vi "Test Process No Process Errors Through Basic Lifecycle.vi"(8 "error in (no error)":errorcluster, 11 "Process Test In":refnum<class "Process Dev Test.lvclass">) -> (0 "error out":errorcluster, 3 "Process Test Out":refnum<class "Process Dev Test.lvclass">)   [LabVIEW 2020, in "Process Dev Test.lvclass"]
uses:
  Mock Error Handler/Mock Error Handler.lvclass
  C:/Git/astemes-triarc-framework/source/Framework/Error Handler Interface/Error Handler Interface.lvclass
  Framework/Process/Process.lvclass/Process.ctl
  <vilib>/Astemes/LUnit/Test Case.lvclass/Test Case.ctl
  <vilib>/Astemes/LUnit/LUnit Assertion Result.lvclass/LUnit Assertion Result.ctl
  <vilib>/Astemes/LUnit/LUnit Test Case Result.lvclass/LUnit Test Case Result.ctl
  <vilib>/Astemes/LUnit/LUnit Method Result.lvclass/LUnit Method Result.ctl
  Framework/Process/Protected/Messaging/Enqueue Message.vi
  Framework/Process/Public/Lifecycle/Get Lifecycle State.vi
  Framework/Process/Private/SubVIs/Wait for finish.vi
  Framework/Process/Private/SubVIs/Set Lifecycle State.vi
  <vilib>/Astemes/LUnit/Palette/Pass.vi
  <vilib>/Astemes/LUnit/Palette/Fail.vi
  <vilib>/Astemes/LUnit/Set Assertion Type.vi
  Framework/Process/Private/SubVIs/Handle Debug Data.vi
  <vilib>/Utility/error.llb/Clear Errors.vi
  <vilib>/Astemes/LUnit/Add test result.vi
  <vilib>/Astemes/LUnit/LUnit Write Passed.vi
  <vilib>/Astemes/LUnit/LUnit Write Message.vi
  <vilib>/Astemes/LUnit/LUnit Write Description.vi
  <vilib>/Astemes/LUnit/LUnit Write Assertion Type.vi
  Framework/Logging/Log Debug.vi
  <vilib>/AdvancedString/1D String Array to Delimited String.vi
  <vilib>/Utility/High Resolution Relative Seconds.vi
  <vilib>/Astemes/LUnit/LUnit Record Assertion Result.vi
  <vilib>/Astemes/LUnit/LUnit Aggregate Assertion Results.vi
  <vilib>/Astemes/LUnit/Assertion Result/LUnit Read Status.vi
  <vilib>/Astemes/LUnit/LUnit Read Message.vi
  <vilib>/Astemes/LUnit/LUnit Read Description.vi
  <vilib>/Astemes/LUnit/Method Result/LUnit Merge Status.vi
  <vilib>/Astemes/LUnit/LUnit Concatenate result strings.vi
  <vilib>/Utility/error.llb/Error Cluster From Error Code.vi
  Framework/Process/Public/Read Name.vi
  <vilib>/Astemes/LUnit/LUnit Assertion Result.lvclass
  Framework/Process/Process.lvclass
  Process Test.lvclass/Process Test.ctl
  tests/Process Development Test/Process Test/Process Dev Test.lvclass
  tests/Process Development Test/Process Test/Process Dev Test.lvclass/Process Dev Test.ctl
  <vilib>/Astemes/LUnit/Test Case.lvclass
  C:/Git/astemes-triarc-framework/source/Framework Test Suite/Base Class Test/Base Test.lvclass
  C:/Program Files (x86)/National Instruments/LabVIEW 2020/vi.lib/Astemes/LUnit/Test Case.lvclass
  C:/Git/astemes-triarc-framework/tests/Process Development Test/Process Test/Process Dev Test.lvclass
  C:/Git/astemes-triarc-framework/source/Framework/Base/Base.lvclass
  C:/Git/astemes-triarc-framework/source/Framework Test Suite/Mock Error Handler/Mock Error Handler.lvclass
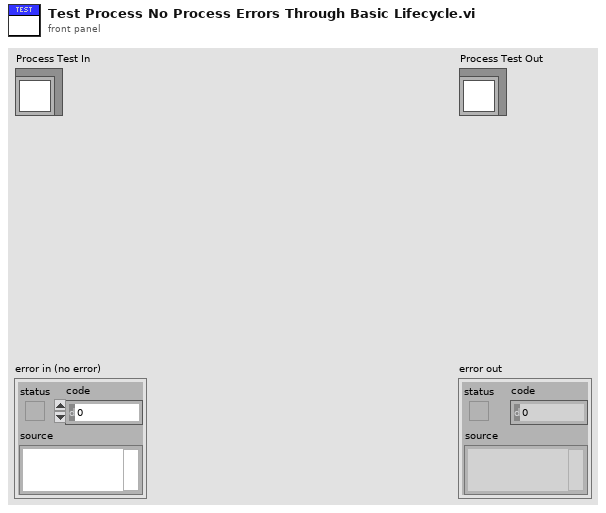
[diagram p1: front panel]
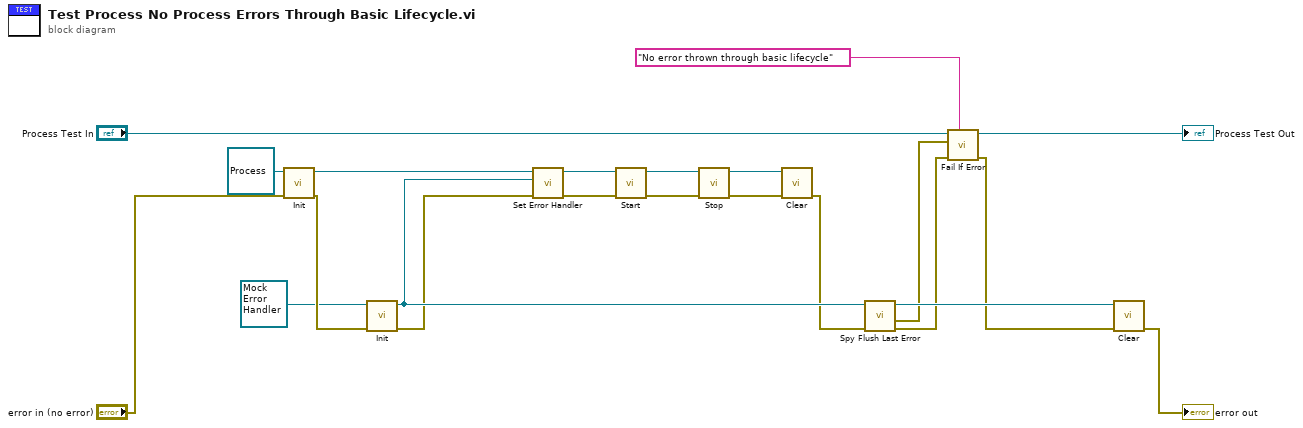
[diagram p0: block diagram]
diagram:
  n1 = call-dynamic "Init.vi"("error in (no error)"="error in (no error)", "Process In"=refnum<class "Process.lvclass"> refnum) -> ("error out"=w22:errorcluster, "Process Out"=w20:refnum<class "Process.lvclass">)  [unwired: 8 in]
  n2 = call-dynamic "Init.vi"("error in (no error)"=w22, "Mock Error Handler In"=refnum<class "Mock Error Handler.lvclass"> refnum ("Mock Error Handler.lvclass")) -> ("error out"=w12:errorcluster, "Mock Error Handler Out"=w13:refnum<class "Mock Error Handler.lvclass">)  [unwired: 8 in]
  n3 = call "Set Error Handler.vi"("error in (no error)"=w12, "Error Handler"=w13, "Process In"=w20) -> ("error out"=w18:errorcluster, "Process Out"=w19:refnum<class "Process.lvclass">)  [unwired: 7 in]
  n4 = call "Start.vi"("error in (no error)"=w18, "Process In"=w19) -> ("error out"=w16:errorcluster, "Process Out"=w17:refnum<class "Process.lvclass">)  [unwired: 7 in, 1 out]
  n5 = call "Stop.vi"("error in (no error)"=w16, "Process In"=w17) -> ("error out"=w14:errorcluster, "Process Out"=w15:refnum<class "Process.lvclass">)  [unwired: 7 in, 1 out]
  n6 = call-dynamic "Clear.vi"("error in (no error)"=w14, "Process In"=w15) -> ("error out"=w9:errorcluster)  [unwired: 9 in]
  n7 = call "Spy Flush Last Error.vi"("error in (no error)"=w9, "Mock Error Handler In"=w13) -> ("error out"=w8:errorcluster, "Error"=w7:errorcluster, "Mock Error Handler Out"=w11:refnum<class "Mock Error Handler.lvclass">)  [unwired: 7 in]
  n8 = call <vilib>:"Fail If Error.vi"("Description"="No error thrown through basic lifecycle", "error in (no error)"=w8, "Assert error"=w7, "LUnit Test Case In"="Process Test In") -> ("error out"=w6:errorcluster, "LUnit Test Case In"=→"Process Test Out":refnum<class "Process Dev Test.lvclass">)  [unwired: 6 in]
  n9 = call-dynamic "Clear.vi"("error in (no error)"=w6, "Mock Process In"=w11) -> ("error out"=→"error out":errorcluster)  [unwired: 9 in]
